vi "DAQmx Self-Test Device.vi"(0 "device in":tag, 11 "error in":errorcluster) -> (15 "error out":errorcluster)   [LabVIEW 2022 SP3]
doc: "Performs a brief test of device resources. If a failure occurs, refer to your device documentation for more information."
uses:
  nilvaiu.dll
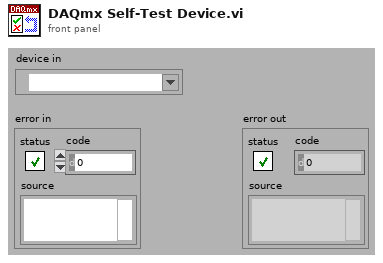
[diagram p1: front panel]
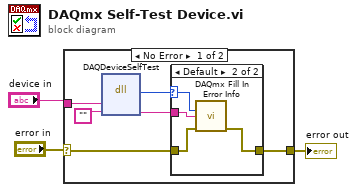
[diagram p0: block diagram]
diagram:
  n1 = case shown="No Error" "error in" {
    selector: "error in" -> [w9 w15]
    tunnel: [w8 w15] -> w3
    tunnel: "device in" -> [w5 _]
    frame No Error {
      n2 = dll-call lib="nilvaiu.*" fn="DAQDeviceSelfTest"("deviceID"=w5, "extendedErrorInfo"="") -> (w7:i32, "extendedErrorInfo"=w6:string)  [unwired: 4 in, 2 out]
      n3 = case shown="Default" w7 {
        selector: w7 -> [_ w12]
        tunnel: w9 -> [w10 w14]
        tunnel: [w10 w13] -> w8
        tunnel: w6 -> [_ w11]
        frame 0 {
        }
        frame Default {
          n4 = call "DAQmx Fill In Error Info.vi"("status code"=w12, "extended error info"=w11, "error in"=w14) -> ("error out"=w13:errorcluster)  [unwired: 1 in, 11 out]
        }
      }
    }
    frame Error {
    }
  }
  "error out" <- w3
